vi "Peregrine_eeprom_read.vi"(0 "Handle in":refnum<visa-resource-name>, 2 "Address":u8, 5 "eeprom address":u32, 11 "error":errorcluster) -> (3 "unsigned byte array":u8[](array[numeric]), 4 "Handle out":refnum<visa-resource-name>, 6 "Key response":u32, 8 "Value response":u32, 15 "error out":errorcluster)   [LabVIEW 2019]
panel:
  out "length":i32
  out "Command":i32
  out "Address response":u8
  # "Inputs"
  # "Response message"
  # "Output"
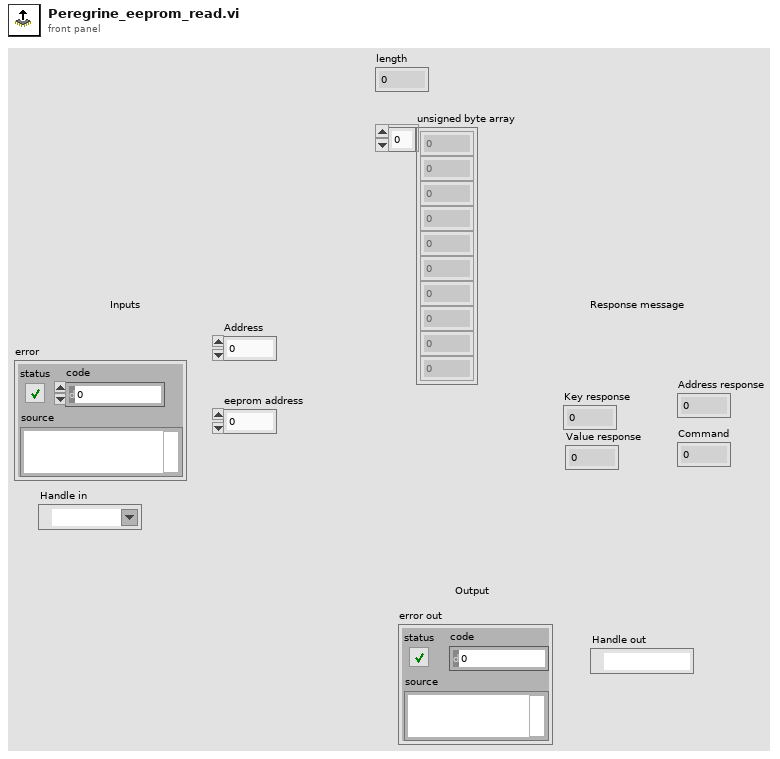
[diagram p1: front panel]
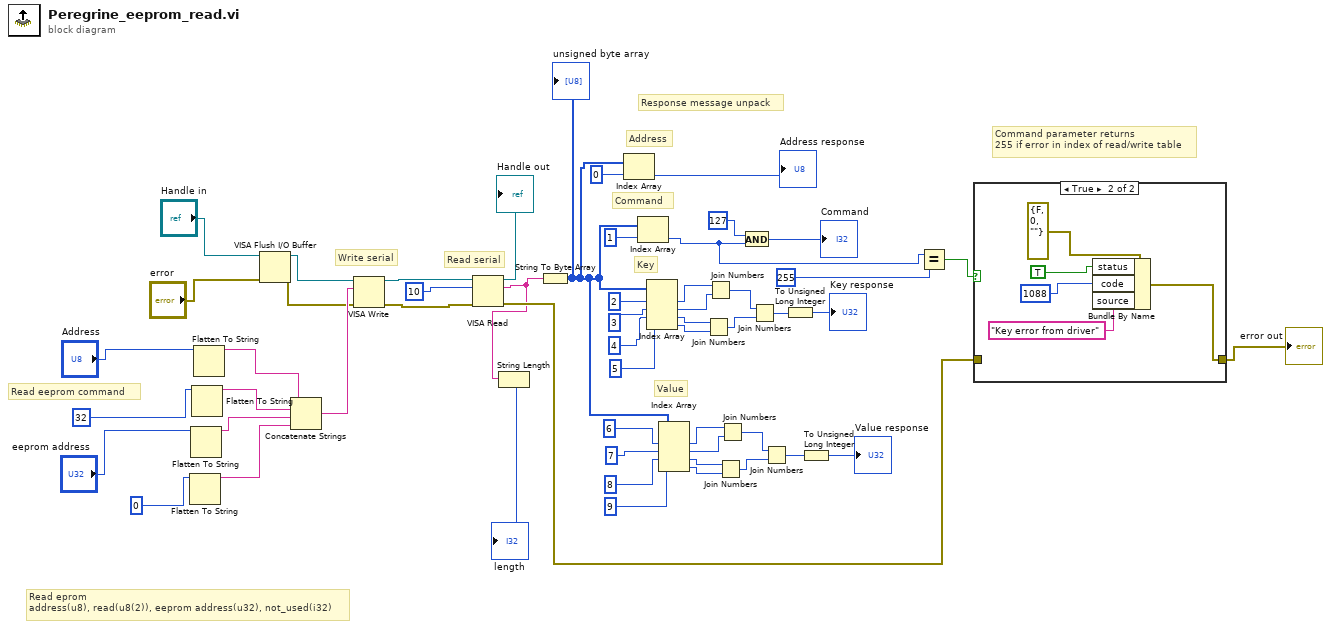
[diagram p0: block diagram]
diagram:
  # "Command parameter returns\n255 if error in index of read/write table"
  # "Value"
  # "Response message unpack"
  # "Read eeprom command"
  # "Command"
  # "Address"
  # "Key"
  # "Read serial"
  # "Write serial"
  # "Read eprom\naddress(u8), read(u8(2)), eeprom address(u32), not_used(i32)"
  n1 = Flatten To String(anything=0) -> (data string=w31:string)  [unwired: 3 in, 2 out]
  n2 = Flatten To String(anything="eeprom address") -> (data string=w32:string)  [unwired: 3 in, 2 out]
  n3 = Flatten To String(anything=u8 32) -> (data string=w10:string)  [unwired: 3 in, 2 out]
  n4 = Flatten To String(anything="Address") -> (data string=w34:string)  [unwired: 3 in, 2 out]
  n5 = VISA Flush I/O Buffer(VISA resource name="Handle in", error in (no error)="error") -> (VISA resource name out=w4:refnum<visa-resource-name>, error out=w3:errorcluster)  [unwired: 1 in]
  n6 = Concatenate Strings(w34, w10, w32, w31) -> (w9:string)
  n7 = VISA Write(VISA resource name=w4, write buffer=w9, error in (no error)=w3) -> (VISA resource name out=w54:refnum<visa-resource-name>, error out=w36:errorcluster)  [unwired: 1 out]
  n8 = VISA Read(VISA resource name=w54, byte count=10, error in (no error)=w36) -> (VISA resource name out=→"Handle out":refnum<visa-resource-name>, read buffer=w2:string, error out=w13:errorcluster)  [unwired: 1 out]
  n9 = String Length(string=w2) -> (length=→"length":i32)
  n10 = String To Byte Array(string=w2) -> (unsigned byte array=w22:u8[])
  "unsigned byte array" <- w22
  n11 = Index Array(array=w22, index=0) -> (element=→"Address response":u8)
  n12 = Index Array(array=w22, index=1) -> (element=w16:u8)
  n13 = Index Array(array=w22, index #1=2, index #2=3, index #3=4, index #4=5) -> (element #1=w46:u8, element #2=w45:u8, element #3=w44:u8, element #4=w43:u8)
  n14 = Index Array(array=w22, index #1=6, index #2=7, index #3=8, index #4=9) -> (element #1=w29:u8, element #2=w28:u8, element #3=w27:u8, element #4=w26:u8)
  n15 = Join Numbers(hi=w44, lo=w43) -> ((hi.lo)=w42:u16)
  n16 = Join Numbers(hi=w46, lo=w45) -> ((hi.lo)=w41:u16)
  n17 = Join Numbers(hi=w27, lo=w26) -> ((hi.lo)=w25:u16)
  n18 = Join Numbers(hi=w29, lo=w28) -> ((hi.lo)=w24:u16)
  n19 = And(x=127, y=w16) -> (x .and. y?=→"Command":i32)
  n20 = Join Numbers(hi=w41, lo=w42) -> ((hi.lo)=w18:u32)
  n21 = Join Numbers(hi=w24, lo=w25) -> ((hi.lo)=w8:u32)
  n22 = To Unsigned Long Integer(number=w18) -> (unsigned 32bit integer=→"Key response":u32)
  n23 = To Unsigned Long Integer(number=w8) -> (unsigned 32bit integer=→"Value response":u32)
  n24 = Equal?(x=w16, y=255) -> (x = y?=w14:bool)
  n25 = case shown="True" w14 {
    tunnel: w13 -> [w55 _]
    tunnel: [w55 w57] -> w12
    frame False {
    }
    frame True {
      n26 = Bundle By Name(cluster=errorcluster {"status"=FALSE, "code"=0, "source"=""} ("error constant"), "status"=TRUE, "code"=1088, "source"="Key error from driver") -> (w57:errorcluster)
    }
  }
  "error out" <- w12
